vi "Delete elements in array.vi"(9 "Elements to Delete":i32[](array[numeric]), 10 "Input Array":variant[](array[variant])) -> (2 "Output Array":variant[](array[variant]))   [LabVIEW 2014, in "Melody Extraction.lvlib"]
uses:
  Melody Extraction.lvlib
panel:
  out "Deleted Elements":variant[](array[variant])
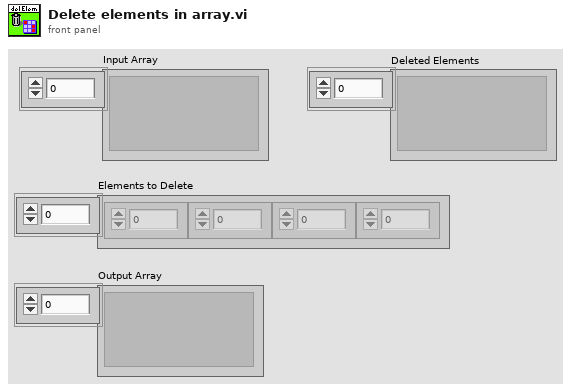
[diagram p1: front panel]
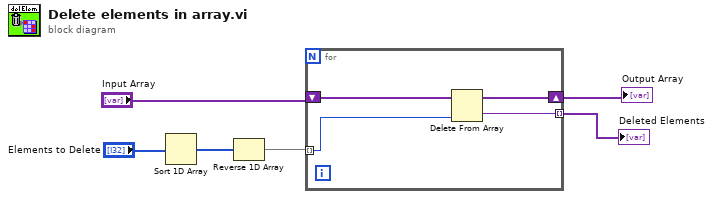
[diagram p0: block diagram]
diagram:
  n1 = Sort 1D Array(array="Elements to Delete") -> (sorted array=w3:i32[])
  n2 = Reverse 1D Array(array=w3) -> (reversed array=w2:i32[])
  n3 = for {
    shift-right: [w9] -> w5
    shift-left: "Input Array" -> [w10]
    tunnel: w2 -> [w8] mode=indexing
    tunnel: [w7] -> w1 mode=indexing
    n4 = Delete From Array(array=w10, index=w8) -> (deleted portion=w7:variant, array with subset deleted=w9:variant[])  [unwired: 1 in]
  }
  "Output Array" <- w5
  "Deleted Elements" <- w1
